vi "Create SetID.vi"(8 "error in (no error)":errorcluster, 10 "ChipID":u8=1, 11 "BML Pattern Creater in":refnum<class "BML Pattern Creater.lvclass">) -> (0 "error out":errorcluster, 2 "Pattern Script All out":string, 3 "BML Pattern Creater out":refnum<class "BML Pattern Creater.lvclass">)   [LabVIEW 2018, in "BML Pattern Creater.lvlib" / "BML Pattern Creater.lvclass"]
uses:
  BML Pattern Creater.lvclass
  Ctls/OM - BML.ctl
  Ctls/RW Options.ctl
  Special Frame.ctl
  Ctls/FRM Data - BML.ctl
  Ctls/Burst Length.ctl
  BML Pattern Creater.lvclass/BML Pattern Creater.ctl
  Write Frame Data.vi
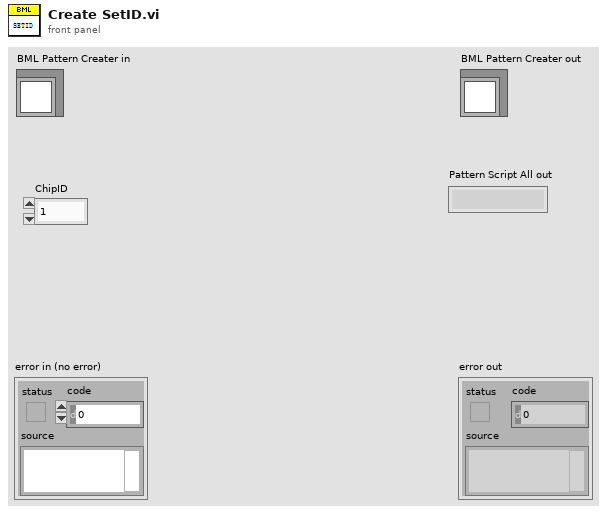
[diagram p1: front panel]
types:
  T1 = typedef "FRM Data - BML.ctl" = cluster{"Pattern_Name":string, "Data":u8[], "Start_Addr":u16, "ChipID":u8, "num of wait ms":i8, "Opcode":string[], "BML OM":T2, "BurstLength":T3, "FSN":u8, "R/W?":T4}
  T2 = typedef "OM - BML.ctl" = enum16{"Normal", "ImmeEffect", "InitSlaveID", "LoadData"}
  T3 = typedef "Burst Length.ctl" = enum8{"0", "2", "3", "4", "5", "8", "16", "32"}
  T4 = typedef "RW Options.ctl" = enum16{"Read", "Write", "R/W"}
  T5 = typedef "BML Pattern Creater.lvlib/BML Pattern Creater.lvclass/Special Frame.ctl" = enum16{"Sync Header", "BML Header", "SW Trig", "SetID State", "Exit SetID State", "SW Reset", "Wait"}
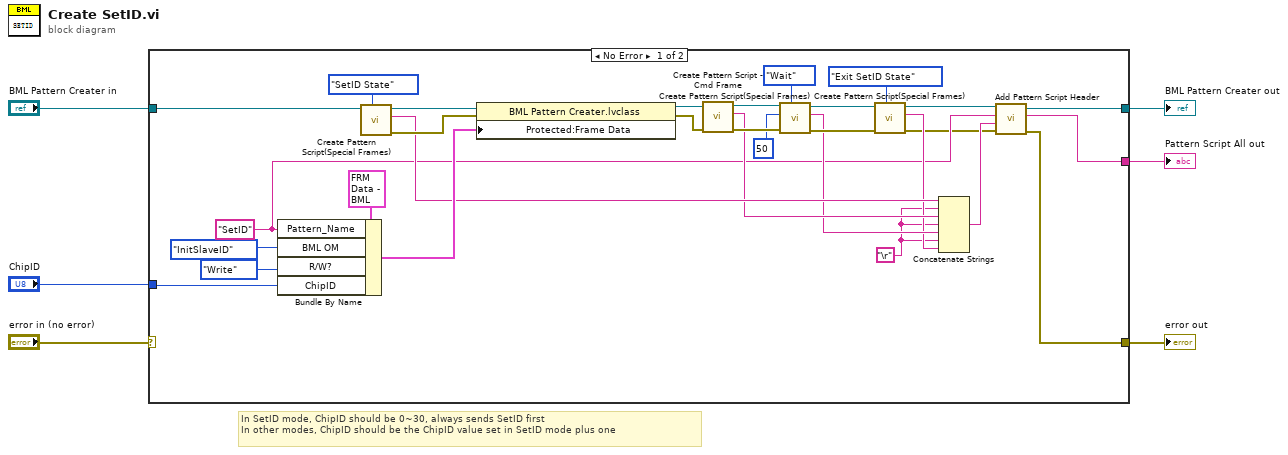
[diagram p0: block diagram]
diagram:
  # "In SetID mode, ChipID should be 0~30, always sends SetID first\nIn other modes, ChipID should be the ChipID value set in SetID mode plus one"
  n1 = case shown="No Error" "error in (no error)" {
    selector: "error in (no error)" -> [_ w38]
    tunnel: [w8 w38] -> w5
    tunnel: [w12 w37] -> w3
    tunnel: "BML Pattern Creater in" -> [w30 w37]
    tunnel: "ChipID" -> [w31 _]
    tunnel: [w7 _] -> w1
    frame No Error {
      w14 = "\r"
      w11 = "SetID" ("Pattern_Name")
      n2 = Bundle By Name(cluster=T1 {"Pattern_Name"="", "Data"=[], "Start_Addr"=0, "ChipID"=1, "num of wait ms"=0, "Opcode"=[], "BML OM"=enum."Normal", "BurstLength"=enum."0", "FSN"=0, "R/W?"=enum."Read"} ("Frame Data"), "Pattern_Name"=w11, "BML OM"=OM_-_BML."InitSlaveID", "R/W?"=RW_Options."Write", "ChipID"=w31) -> (w34:T1)
      n3 = call "Create Pattern Script(Special Frames).vi"("Special Frame Type"=Special_Frame."SetID State", "BML Pattern Creater in"=w30) -> ("error out"=w28:errorcluster, "string out"=w18:string, "BML Pattern Creater out"=w29:refnum<class "BML Pattern Creater.lvclass">)  [unwired: 7 in]
      n4 = property class="BML Pattern Creater.lvclass"(reference=w29, error in=w28, "Protected:Frame Data"=w34) -> (reference out=w33:refnum<class "BML Pattern Creater.lvclass">, error out=w32:errorcluster)
      n5 = call "Create Pattern Script - Cmd Frame.vi"("error in (no error)"=w32, "BML Pattern Creater in"=w33) -> ("error out"=w25:errorcluster, "CMD Frame out"=w17:string, "BML Pattern Creater out"=w26:refnum<class "BML Pattern Creater.lvclass">)  [unwired: 7 in]
      n6 = call "Create Pattern Script(Special Frames).vi"("Special Frame Type"=Special_Frame."Wait", "error in (no error)"=w25, "Num of Timeset"=u32 50, "BML Pattern Creater in"=w26) -> ("error out"=w21:errorcluster, "string out"=w16:string, "BML Pattern Creater out"=w22:refnum<class "BML Pattern Creater.lvclass">)  [unwired: 5 in]
      n7 = call "Create Pattern Script(Special Frames).vi"("Special Frame Type"=Special_Frame."Exit SetID State", "error in (no error)"=w21, "BML Pattern Creater in"=w22) -> ("error out"=w9:errorcluster, "string out"=w15:string, "BML Pattern Creater out"=w13:refnum<class "BML Pattern Creater.lvclass">)  [unwired: 6 in]
      n8 = Concatenate Strings(w18, w14, w17, w14, w16, w14, w15) -> (w10:string)
      n9 = call "Add Pattern Script Header.vi"("error in (no error)"=w9, "Pattern Script Frame in"=w10, "Pattern Name"=w11, "BML Pattern Creater"=w13) -> ("error out"=w8:errorcluster, "Pattern Script All out"=w7:string, "BML Pattern Creater"=w12:refnum<class "BML Pattern Creater.lvclass">)  [unwired: 5 in]
    }
    frame Error {
    }
  }
  "error out" <- w5
  "BML Pattern Creater out" <- w3
  "Pattern Script All out" <- w1
